vi "Enable Loads.vi"(8 "error in (no error)":errorcluster, 11 "Driver Test in":refnum<class "Driver Test.lvclass">) -> (0 "error out":errorcluster)   [LabVIEW 2015, in "Driver Test.lvclass"]
doc: "Sets the DC Loads into their Run State."
uses:
  Driver Test.lvclass
  CBTF Applications/Driver Board Testing/Main/Application/Application/Class/typedefs/Instrument Selector -- Enum.ctl
  Classes/Instruments/DC Load/DC Load/Class/DC Load.lvclass
  Test Class/Test Class.lvclass
  Classes/Application/Class/Application.lvclass
  CBTF Applications/Driver Board Testing/Main/Application/Application/Class/Driver Board Test.lvclass
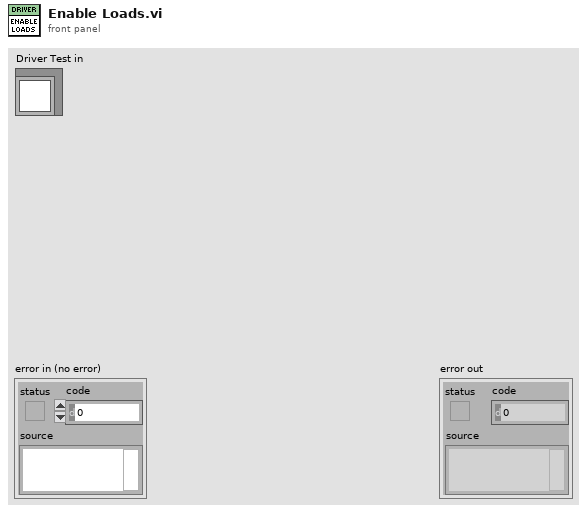
[diagram p1: front panel]
types:
  T1 = typedef "Driver Board Test.lvlib/Driver Board Test.lvclass/Instrument Selector -- Enum.ctl" = enum16{"ACPS1", "ACPS2", "DCPS1", "DCPS2", "DCPS3", "DCLoad1", "DCLoad2", "DPM1", "DPM2", "Switch1", "PXI1Slot2", "PXI1Slot3", "cDAQ1Mod5", "cDAQ1Mod6", "cDAQ1Mod7", "cDAQ1Mod8", "cDAQ1Mod1", "cDAQ1Mod2", "cDAQ1Mod3", "cDAQ1Mod4", "cDAQ2Mod1", "cDAQ2Mod2", "cDAQ2Mod3", "cDAQ2Mod4"}
  T2 = typedef "Application.lvlib/App Properties.lvclass/Class Properties -- Cluster.ctl" = cluster{"UUT Info":T3[], "Test Information":refnum<vi>, "Shop Floor System":refnum<class "Shop Floor System.lvclass">, "Gold Board":refnum<class "Golden Board.lvclass">, "Test Recipe":refnum<class "Test Recipe.lvclass">, "Instruments":refnum<class "Instrument.lvclass">[], "Mode":T4, "Test Results":T5[], "Station Config":refnum<class "Station Config.lvclass">, "Variable Engine":refnum<class "Variable Engine.lvclass">}
  T3 = typedef "Application.lvlib/App Properties.lvclass/UUT Reference -- Cluster.ctl" = cluster{"Serial Number Reference":refnum<vi>, "Status Message Reference":refnum<vi>}
  T4 = typedef "Application.lvlib/Application.lvclass/Op Mode -- Enum.ctl" = u16
  T5 = typedef "Application.lvlib/App Properties.lvclass/Test Result -- Cluster.ctl" = cluster{"Position":i32, "Pass":bool, "Fail Codes":string}
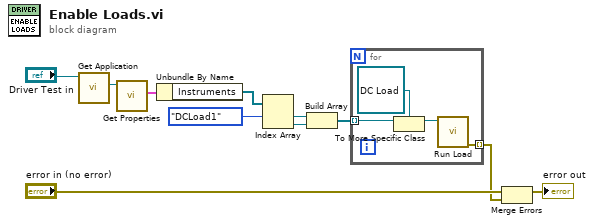
[diagram p0: block diagram]
diagram:
  n1 = call "Get Application.vi"("Test Class in"="Driver Test in") -> ("Application.lvlib:Application.lvclass"=w7:refnum<class "Application.lvclass">)  [unwired: 9 in, 1 out]
  n2 = call "Get Properties.vi"("Acrobat Template in"=w7) -> ("Class Properties"=w8:T2)  [unwired: 8 in, 2 out]
  n3 = Unbundle By Name(w8) -> ("Instruments"=w5:refnum<class "Instrument.lvclass">[])
  n4 = Index Array(array=w5, index #1=Instrument_Selector_--_Enum."DCLoad1" ("Instrument")) -> (element #1=w4:refnum<class "Instrument.lvclass">, element #2=w3:refnum<class "Instrument.lvclass">)  [unwired: 1 in]
  n5 = Build Array(w4, w3) -> (w2:refnum<class "Instrument.lvclass">[])
  n6 = for {
    tunnel: w2 -> [w14] mode=indexing
    tunnel: [w12] -> w1 mode=indexing
    n7 = To More Specific Class(target class=refnum<class "DC Load.lvclass"> refnum ("DC Load out"), reference=w14) -> (specific class reference=w13:refnum<class "DC Load.lvclass">)  [unwired: 1 in, 1 out]
    n8 = call-dynamic "Run Load.vi"("DC Load in"=w13) -> ("error out"=w12:errorcluster)  [unwired: 9 in, 1 out]
  }
  n9 = Merge Errors("error in (no error)", w1) -> (→"error out":errorcluster)
